vi "RemoveTails (SubVI).vi"(7 "Side of Tail":T1=enum."Left tail", 8 "error in (no error)":errorcluster, 9 "delta y values":dbl[](array[numeric]), 10 "y values":dbl[](array[numeric]), 11 "x values":dbl[](array[numeric])) -> (0 "error out":errorcluster, 1 "Selected delta y values":dbl[](array[numeric]), 2 "Selected y values":dbl[](array[numeric]), 3 "Selected x values":dbl[](array[numeric]))   [LabVIEW 2016]
doc: "This VI removes a tail on the left or \nright hand sides of a dataset."
uses:
  Utils/Enum_TypeDefinitions/Enum_TypeDef_Tails.ctl
  <vilib>/Analysis/baseanly.llb/Mean (DBL).vi
  <vilib>/measure/mascope.llb/Transition Measurements 1 chan.vi
  <vilib>/measure/NI_MAPro.lvlib
  <vilib>/Analysis/NI_AALBase.lvlib
panel:
  # "This VI removes a tail on the left or \nright hand sides of a dataset."
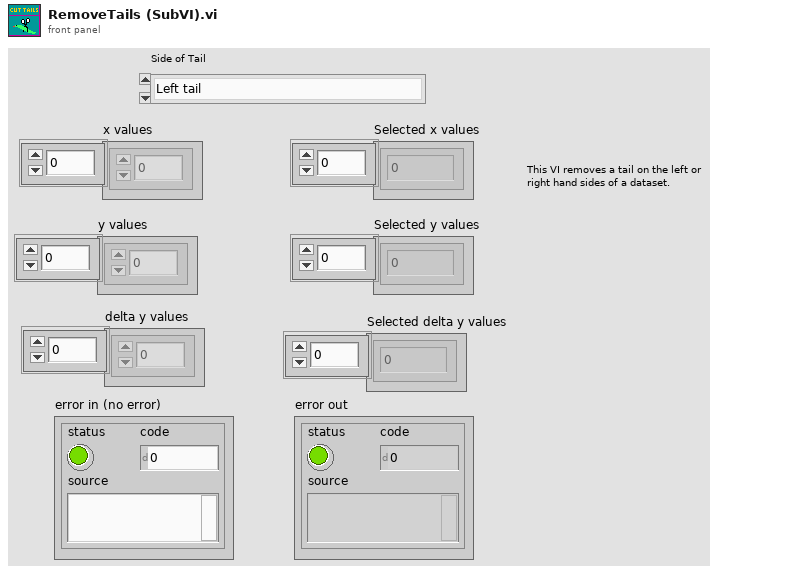
[diagram p1: front panel]
types:
  T1 = typedef "Enum_TypeDef_Tails.ctl" = enum16{"No tails", "Left tail", "Right tail"}
  T2 = cluster{"high ref level":dbl, "mid ref level":dbl, "low ref level":dbl, "ref units":u16}
  T3 = cluster{"start time":dbl, "end time":dbl, "ref levels":cluster{"high ref level":dbl, "mid ref level":dbl, "low ref level":dbl, "ref units":u16}}
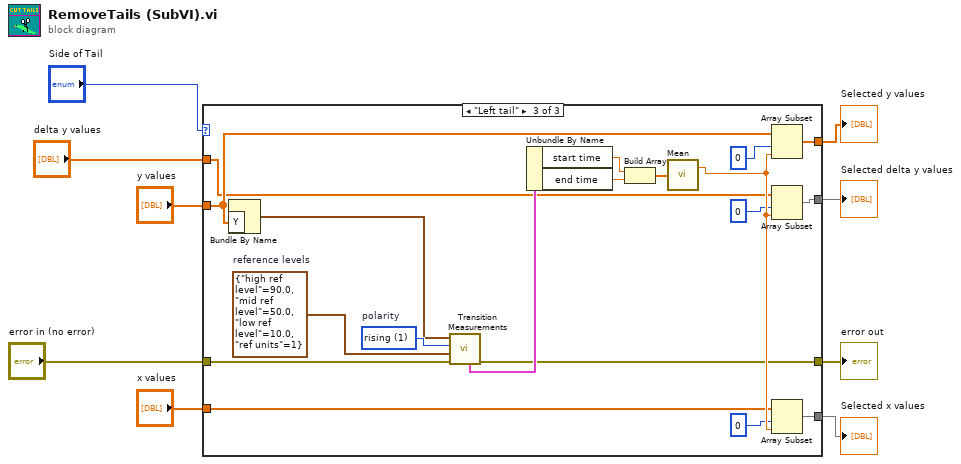
[diagram p0: block diagram]
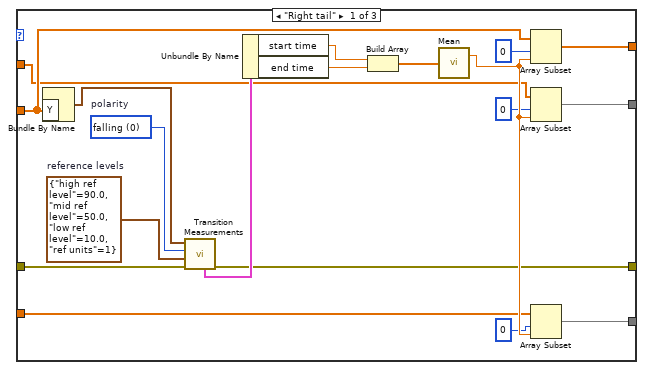
[diagram p2: hidden frame]
diagram:
  n1 = case shown="\"Left tail\"" "Side of Tail" {
    tunnel: "y values" -> [w17 w31 w40]
    tunnel: "x values" -> [w16 w32 w39]
    tunnel: "error in (no error)" -> [w11 w29 w38]
    tunnel: "delta y values" -> [w13 w30 w37]
    tunnel: [w12 w30 w36] -> w4
    tunnel: [w14 w31 w35] -> w3
    tunnel: [w15 w32 w34] -> w2
    tunnel: [w10 w29 w33] -> w1
    frame "Right tail" {
      w28 = u16 0 items=["falling", "rising"]  # polarity
      w26 = T2 {"high ref level"=90.0, "mid ref level"=50.0, "low ref level"=10.0, "ref units"=1}  # reference levels
      n2 = Bundle By Name("Y"=w17) -> (w21:waveform(dbl))  [unwired: 1 in]
      n3 = call-poly <vilib>:"Transition Measurements.vi"("error in (no error)"=w11, "reference levels"=w26, "polarity (rising)"=w28, "signal in"=w21) -> ("error out"=w10:errorcluster, "measurement info"=w22:T3)  [unwired: 2 in, 4 out]
      n4 = Unbundle By Name(w22) -> ("start time"=w18:dbl, "end time"=w19:dbl)
      n5 = Build Array(w18, w19) -> (w20:dbl[])
      n6 = call-poly <vilib>:"Mean.vi"("X"=w20) -> ("mean"=w27:dbl)  [unwired: 1 out]
      n7 = Array Subset(array=w17, index=0, length=w27) -> (w14:dbl[])
      n8 = Array Subset(array=w13, index=0, length=w27) -> (w12:dbl[])
      n9 = Array Subset(array=w16, index=0, length=w27) -> (w15:dbl[])
    }
    frame "No tails", Default {
    }
    frame "Left tail" {
      w51 = u16 1 items=["falling", "rising"]  # polarity
      w49 = T2 {"high ref level"=90.0, "mid ref level"=50.0, "low ref level"=10.0, "ref units"=1}  # reference levels
      n10 = Bundle By Name("Y"=w40) -> (w44:waveform(dbl))  [unwired: 1 in]
      n11 = call-poly <vilib>:"Transition Measurements.vi"("error in (no error)"=w38, "reference levels"=w49, "polarity (rising)"=w51, "signal in"=w44) -> ("error out"=w33:errorcluster, "measurement info"=w45:T3)  [unwired: 2 in, 4 out]
      n12 = Unbundle By Name(w45) -> ("start time"=w41:dbl, "end time"=w42:dbl)
      n13 = Build Array(w41, w42) -> (w43:dbl[])
      n14 = call-poly <vilib>:"Mean.vi"("X"=w43) -> ("mean"=w50:dbl)  [unwired: 1 out]
      n15 = Array Subset(array=w40, index=0, length=w50) -> (w35:dbl[])
      n16 = Array Subset(array=w37, index=0, length=w50) -> (w36:dbl[])
      n17 = Array Subset(array=w39, index=0, length=w50) -> (w34:dbl[])
    }
  }
  "Selected delta y values" <- w4
  "Selected y values" <- w3
  "Selected x values" <- w2
  "error out" <- w1
